vi "Statusword.vi"(11 "Wert":u16) -> (2 "Status":T1(ring))   [LabVIEW 2014]
uses:
  Statusword.ctl
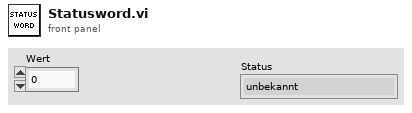
[diagram p1: front panel]
types:
  T1 = enum16{"unbekannt", "Quick stop active", "Fault reaction active", "Fault", "Operation enabled", "Switched on", "Ready to switch on", "Switch on disabled", "Not Ready to switch on"}
  T2 = typedef "Statusword.ctl" = enum16{"unbekannt", "Quick stop active", "Fault reaction active", "Fault", "Operation enabled", "Switched on", "Ready to switch on", "Switch on disabled", "Not Ready to switch on"}
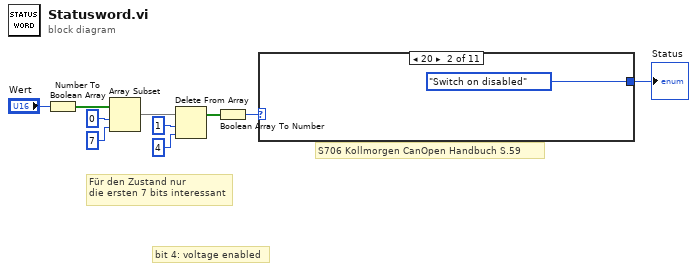
[diagram p0: block diagram]
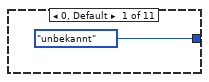
[diagram p2: hidden frame]
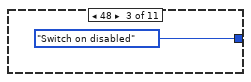
[diagram p3: hidden frame]
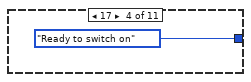
[diagram p4: hidden frame]
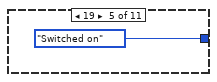
[diagram p5: hidden frame]
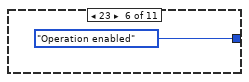
[diagram p6: hidden frame]
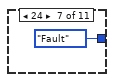
[diagram p7: hidden frame]
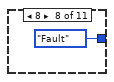
[diagram p8: hidden frame]
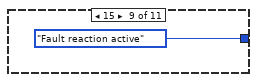
[diagram p9: hidden frame]
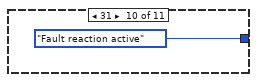
[diagram p10: hidden frame]
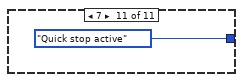
[diagram p11: hidden frame]
diagram:
  # "S706 Kollmorgen CanOpen Handbuch S.59"
  # "bit 4: voltage enabled"
  # "Für den Zustand nur\ndie ersten 7 bits interessant"
  n1 = Number To Boolean Array(number="Wert") -> (Boolean array=w9:bool[])
  n2 = Array Subset(array=w9, index=0 ("Index"), length=7 ("Länge")) -> (w5:bool[])
  n3 = Delete From Array(array=w5, length=1 ("Länge"), index=4 ("Index")) -> (array with subset deleted=w4:bool[])  [unwired: 1 out]
  n4 = Boolean Array To Number(Boolean array=w4) -> (number=w6:u32)
  n5 = case shown="20" w6 {
    tunnel: [Statusword."unbekannt" ("Status") Statusword."Switch on disabled" ("Status") Statusword."Switch on disabled" ("Status") Statusword."Ready to switch on" ("Status") Statusword."Switched on" ("Status") Statusword."Operation enabled" ("Status") Statusword."Fault" ("Status") Statusword."Fault" ("Status") Statusword."Fault reaction active" ("Status") Statusword."Fault reaction active" ("Status") Statusword."Quick stop active" ("Status")] -> w1
    frame 0, Default {
    }
    frame 32 {
    }
    frame 48 {
    }
    frame 17 {
    }
    frame 19 {
    }
    frame 23 {
    }
    frame 24 {
    }
    frame 8 {
    }
    frame 15 {
    }
    frame 31 {
    }
    frame 7 {
    }
  }
  "Status" <- w1
